vi "Send Simulated P2P FIFO to AI Loop.vi"(4 "NoOfSamples":u16, 5 "LastIterration":bool, 6 "SensorID":u16, 7 "FirstIterration":bool, 8 "ActiveLedIndex":u16, 10 "SendAiCMD":u16, 11 "TimingCounter":u16) -> ()   [LabVIEW 2015]
uses:
  <vilib>/rvi/DataTransferAndStorage/Container/XNode/niFpgaContainer.xnode
  <vilib>/rvi/FIFO/Fifo_Resource/nirvififoEmulationWrite.vi
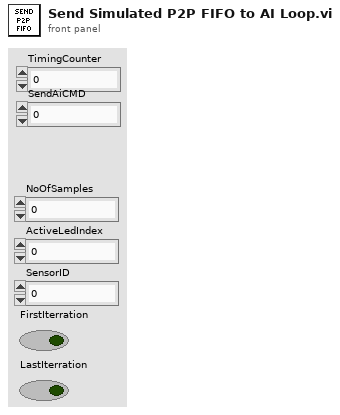
[diagram p1: front panel]
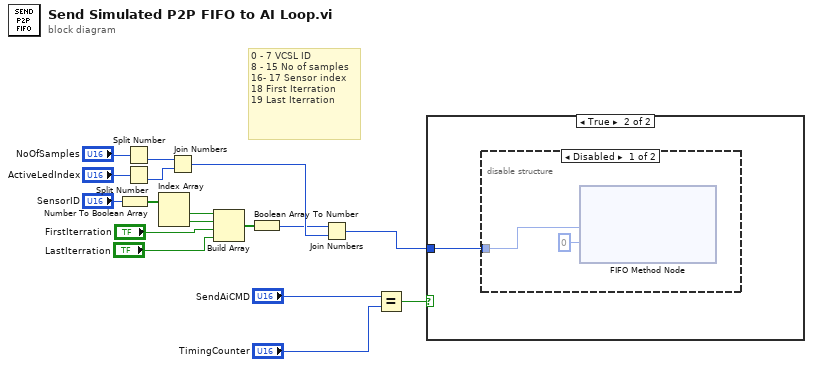
[diagram p0: block diagram]
diagram:
  # "0 - 7 VCSL ID\n8 - 15 No of samples\n16- 17 Sensor index\n18 First Iterration\n19 Last Iterration"
  n1 = Number To Boolean Array(number="SensorID") -> (Boolean array=w8:bool[])
  n2 = Split Number(x="NoOfSamples") -> (lo(x)=w12:u8)  [unwired: 1 out]
  n3 = Split Number(x="ActiveLedIndex") -> (lo(x)=w11:u8)  [unwired: 1 out]
  n4 = Index Array(array=w8) -> (element #1=w7:bool, element #2=w6:bool)  [unwired: 2 in]
  n5 = Join Numbers(hi=w12, lo=w11) -> ((hi.lo)=w3:u16)
  n6 = Build Array(w7, w6, "FirstIterration", "LastIterration") -> (w2:bool[])
  n7 = Boolean Array To Number(Boolean array=w2) -> (number=w1:u16)
  n8 = Join Numbers(hi=w1, lo=w3) -> ((hi.lo)=w14:u32)
  n9 = Equal?(x="SendAiCMD", y="TimingCounter") -> (x = y?=w17:bool)
  n10 = case shown="True" w17 {
    tunnel: w14 -> [_ w18]
    frame False {
    }
    frame True {
      n11 = disable-structure shown="Disabled" {
        disable-tunnel: w18 -> [w20 _]
        frame Disabled {
          n12 = xnode ("FIFO Method Node")("Element"=w20, "Timeout"=0) -> ()  [unwired: 1 in, 2 out]
        }
        frame Enabled {
        }
      }
    }
  }
